vi "WindowsBoundsToRect.vi"(11 "Windows Bounds":T1) -> (3 "Rectangle":T2)   [LabVIEW 2012]
doc: "Computes the Rectangle from the Front Panel Windows Bounds."
uses:
  <vilib>/Utility/miscctls.llb/LVRectTypeDef.ctl
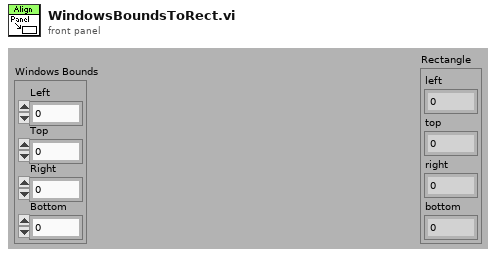
[diagram p1: front panel]
types:
  T1 = typedef "LVRectTypeDef.ctl" = cluster{"Left":i16, "Top":i16, "Right":i16, "Bottom":i16}
  T2 = cluster{"left":i16, "top":i16, "right":i16, "bottom":i16}
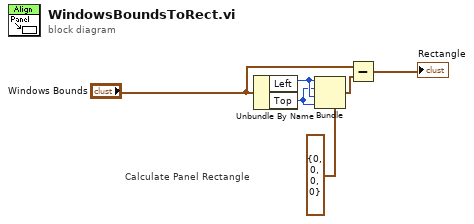
[diagram p0: block diagram]
diagram:
  # "Calculate Panel Rectangle"
  n1 = Unbundle By Name("Windows Bounds") -> ("Left"=w6:i16, "Top"=w5:i16)
  n2 = Bundle(cluster=T2 {"left"=0, "top"=0, "right"=0, "bottom"=0} ("Rectangle"), "left"=w6, "top"=w5, "right"=w6, "bottom"=w5) -> (w4:T2)
  n3 = Subtract(x="Windows Bounds", y=w4) -> (x-y=→"Rectangle":T1)
